vi "Init_Test.vi"(8 "error in (no error)":errorcluster caption="entrée d'erreur (pas d'erreur)", 11 "Test (Default) en entrée":refnum<class "Sequencer (Default).lvclass">) -> (0 "error out":errorcluster caption="sortie d'erreur", 3 "Test (Default) en sortie":refnum<class "Sequencer (Default).lvclass">)   [LabVIEW 2020, in "Library Core.lvlib" / "Sequencer (Default).lvclass"]
uses:
  Sequencer (Default).lvclass
  Sequencer (Default).lvclass/Sequencer (Default).ctl
  Commun VI/TypeDef/Variable Printable.ctl
  Commun VI/TypeDef/Commande Test/Commande Data Test.ctl
  Commun VI/TypeDef/Commande Test/Commande Value Type.ctl
  Commun VI/TypeDef/Commande Test/Commande Type Test.ctl
  Commun VI/TypeDef/Actor Type.ctl
  Launch_Sequencer.vi
  <vilib>/Utility/config.llb/Read Key (String).vi
  Commun VI/Library Commun.lvlib
  <vilib>/Utility/config.llb/NI_LVConfig.lvlib
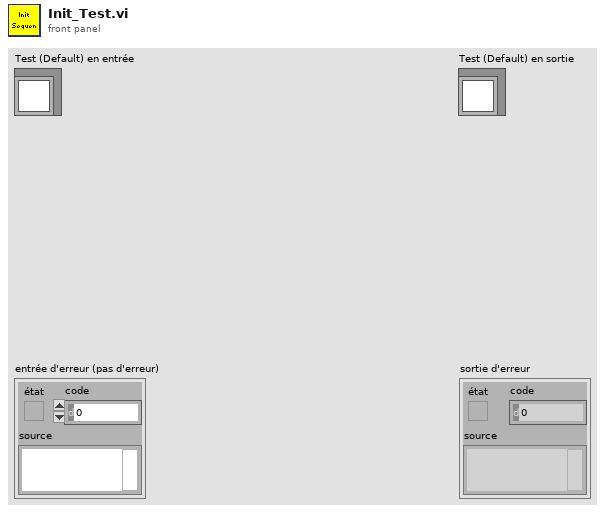
[diagram p1: front panel]
types:
  T1 = enum16{"Get Variable", "Get All Variables", "Set Variable", "Delete Variable", "Delete All Variable"}
  T2 = typedef "Variable Printable.ctl" = string
  T3 = enum16{"Add Instr", "Remove Instr", "List Instr", "Get Instr Class", "Get Instr obj", "Save Insrt obj", "Modify Insrt obj", "Init"}
  T4 = typedef "Library Commun.lvlib/Actor Type.ctl" = enum16{"Default", "Firebase", "Database"}
  T5 = typedef "Library Commun.lvlib/Commande Data Test.ctl" = cluster{"Main Test":string, "Name Test":string, "StartOfTest":string, "Value":string, "Limit_Low":string, "Limit_High":string, "Result":bool, "Fatal_Test":bool, "NbRetry":dbl, "EndOfTest":string, "Error":string, "TypeValue":T6, "Type Test":T7}
  T6 = typedef "Library Commun.lvlib/Commande Value Type.ctl" = enum16{"None", "String", "Number", "Timestamp", "Boolean", "Array"}
  T7 = typedef "Library Commun.lvlib/Commande Type Test.ctl" = enum16{"Function", "Test", "Calculation"}
  T8 = typedef "NI_LVConfig.lvlib/Config Data RefNum.ctl" = refnum<k1>
  T9 = cluster{"Group Name":string, "Tab Test":cluster{"Type Function":string, "Test Name":string, "Class launched by the actors ":string, "Name_Instrument":string, "Class_Instrument":string, "Parameter (Json)":string, "Limit_Low":string, "Limit_Hight":string, "Fatal Test ?":bool, "Parallelized ?":bool, "Mandatory ?":bool}[], "Parallelized ?":bool, "Mandatory ?":bool}[]
  T10 = cluster{"Name":string, "Instrument":refnum<class "Class Instrument (Default).lvclass">, "Close After Autotest":bool}[]
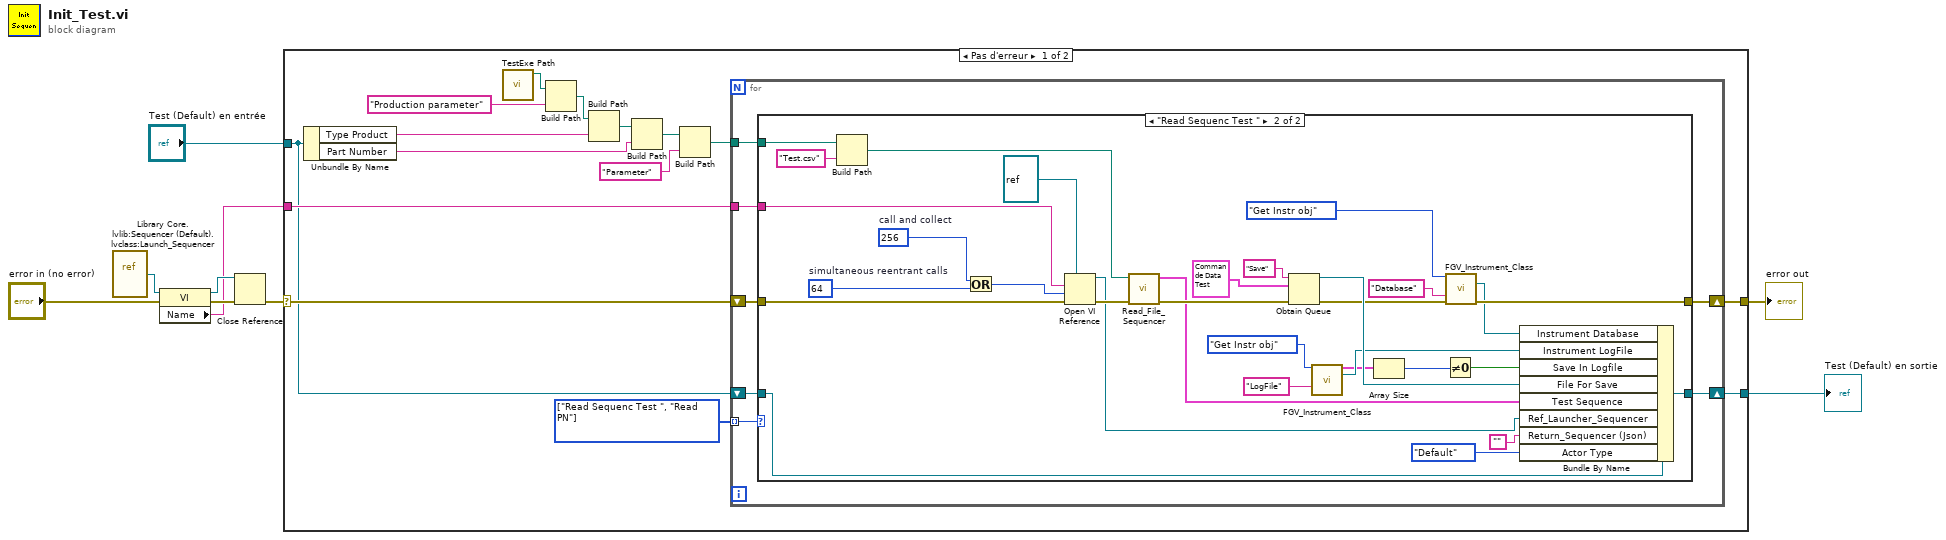
[diagram p0: block diagram]
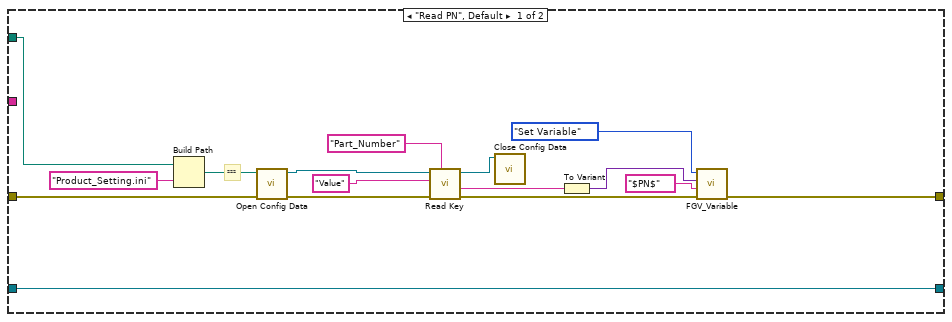
[diagram p2: hidden frame]
diagram:
  n1 = vi-ref "Library Core.lvlib:Sequencer (Default).lvclass:Launch_Sequencer.vi"() -> (w2:refnum<vi>)
  n2 = property class="VI"(reference=w2, error in="error in (no error)") -> (reference out=w9:refnum<vi>, error out=w8:errorcluster, "Name"=w7:string)
  n3 = Close Reference(reference=w9, error in (no error)=w8) -> (error out=w6:errorcluster)
  n4 = case shown="Pas d'erreur" w6 {
    selector: w6 -> [w24 w80]
    tunnel: [w12 w80] -> w1
    tunnel: [w11 w79] -> w4
    tunnel: "Test (Default) en entrée" -> [w15 w79]
    tunnel: w7 -> [w23 _]
    frame No Error {
      w10 = enum16{"Read PN", "Read Sequenc Test "}[] [enum."Read Sequenc Test ", enum."Read PN"] items=["Read PN", "Read Sequenc Test "]
      n5 = Unbundle By Name(w15) -> ("Type Product"=w13:string, "Part Number"=w14:string)
      n6 = call "TestExe Path.vi"() -> ("Chemin Actuel"=w17:path)  [unwired: 9 in, 2 out]
      n7 = Build Path(base path=w17, name or relative path="Production parameter" ("nom ou chemin relatif")) -> (appended path=w20:path)
      n8 = Build Path(base path=w20, name or relative path=w13) -> (appended path=w21:path)
      n9 = Build Path(base path=w21, name or relative path=w14) -> (appended path=w22:path)
      n10 = Build Path(base path=w22, name or relative path="Parameter" ("nom ou chemin relatif")) -> (appended path=w16:path)
      n11 = for {
        tunnel: w23 -> [w30]
        tunnel: w16 -> [w29]
        shift-right: [w27] -> w12
        shift-left: w24 -> [w31]
        shift-right: [w26] -> w11
        shift-left: w15 -> [w28]
        tunnel: w10 -> [w25] mode=indexing
        n12 = case shown="\"Read Sequenc Test \"" w25 {
          tunnel: w31 -> [w37 w78]
          tunnel: w30 -> [_ w77]
          tunnel: w29 -> [w32 w76]
          tunnel: w28 -> [w36 w75]
          tunnel: [w33 w74] -> w27
          tunnel: [w36 w73] -> w26
          frame "Read PN", Default {
            # "²²²"
            n13 = Build Path(base path=w32, name or relative path="Product_Setting.ini" ("nom ou chemin relatif")) -> (appended path=w41:path)
            n14 = call <vilib>:"Open Config Data.vi"("error in (no error)"=w37, "configuration file path"=w41) -> ("error out"=w39:errorcluster, "refnum"=w38:T8)  [unwired: 7 in, 1 out]
            n15 = call-poly <vilib>:"Read Key.vi"("section"="Part_Number" ("nom ou chemin relatif"), "error in (no error)"=w39, "key"="Value", "refnum"=w38) -> ("error out"=w34:errorcluster, "value"=w35:string, "refnum out"=w40:T8)  [unwired: 4 in, 1 out]
            n16 = call <vilib>:"Close Config Data.vi"("refnum"=w40) -> ()  [unwired: 9 in, 2 out]
            n17 = To Variant(anything=w35) -> (Variant=w47:variant)
            n18 = call "FGV_Variable.vi"("error in (no error)"=w34, "Variable"=T2 "$PN$" ("Variable Printable"), "Data In"=w47, "Function"=T1."Set Variable") -> ("error out"=w33:errorcluster)  [unwired: 5 in, 2 out]
          }
          frame "Read Sequenc Test " {
            w71 = 64  # simultaneous reentrant calls
            w70 = 256  # call and collect
            n19 = Build Path(base path=w76, name or relative path="Test.csv" ("nom ou chemin relatif")) -> (appended path=w65:path)
            n20 = Or(x=w70, y=w71) -> (x .or. y?=w69:i32)
            n21 = Open VI Reference(type specifier VI Refnum (for type only)=refnum<vi> refnum ("spécificateur de type du refnum de VI (pour type seulement)"), vi path=w77, options=w69, error in (no error)=w78) -> (vi reference=w56:refnum<vi>, error out=w67:errorcluster)  [unwired: 2 in]
            n22 = call "Read_File_Sequencer.vi"("error in (no error)"=w67, "file path (dialog if empty)"=w65) -> ("error out"=w62:errorcluster, "Test Sequence"=w57:T9)  [unwired: 8 in]
            n23 = Obtain Queue(name (unnamed)="Save" ("nom (aucun)"), element data type=T5 {"Main Test"="", "Name Test"="", "StartOfTest"="", "Value"="", "Limit_Low"="", "Limit_High"="", "Result"=FALSE, "Fatal_Test"=FALSE, "NbRetry"=1.0, "EndOfTest"="", "Error"="", "TypeValue"=enum."None", "Type Test"=enum."Function"} ("Data Test"), error in (no error)=w62) -> (queue out=w61:refnum<queue>, error out=w59:errorcluster)  [unwired: 2 in, 1 out]
            n24 = call "FGV_Instrument_Class.vi"("Action"=T3."Get Instr obj", "Instr name"="LogFile") -> ("Instruments 2"=w52:T10, "Familly class Out"=w54:refnum<class "Class Instrument (Default).lvclass">)  [unwired: 11 in, 1 out]
            n25 = Array Size(array=w52) -> (size(s)=w51:i32)
            n26 = Not Equal To 0?(x=w51) -> (x != 0?=w50:bool)
            n27 = call "FGV_Instrument_Class.vi"("Action"=T3."Get Instr obj", "Instr name"="Database", "error in (no error)"=w59) -> ("Familly class Out"=w53:refnum<class "Class Instrument (Default).lvclass">, "error out"=w74:errorcluster)  [unwired: 10 in, 1 out]
            n28 = Bundle By Name(cluster=w75, "Instrument Database"=w53, "Instrument LogFile"=w54, "Save In Logfile"=w50, "File For Save"=w61, "Test Sequence"=w57, "Ref_Launcher_Sequencer"=w56, "Return_Sequencer (Json)"="" ("Data Test.Error"), "Actor Type"=Actor_Type."Default") -> (w73:refnum<class "Sequencer (Default).lvclass">)
          }
        }
      }
    }
    frame Error {
    }
  }
  "error out" <- w1
  "Test (Default) en sortie" <- w4
